vi "SS Class Init.vi"(7 "VI Refnum":refnum<vi>, 8 "error in (no error)":errorcluster, 9 "Init Data":variant, 10 "Device":string, 11 "Telescope in":refnum<class "Subsystem Telescope.lvclass">) -> (0 "error out":errorcluster, 2 "Channel List":refnum<class "HK Item.lvclass">[](array[class]), 3 "Telescope out":refnum<class "Subsystem Telescope.lvclass">)   [LabVIEW 2024, in "Subsystem Telescope.lvclass"]
uses:
  Subsystem Telescope.lvclass
  hk-channel-class/hk-channel-class/HK Item/HK Item.lvclass
  Subsystem Class.lvclass
  Telescope/Telescope.lvclass
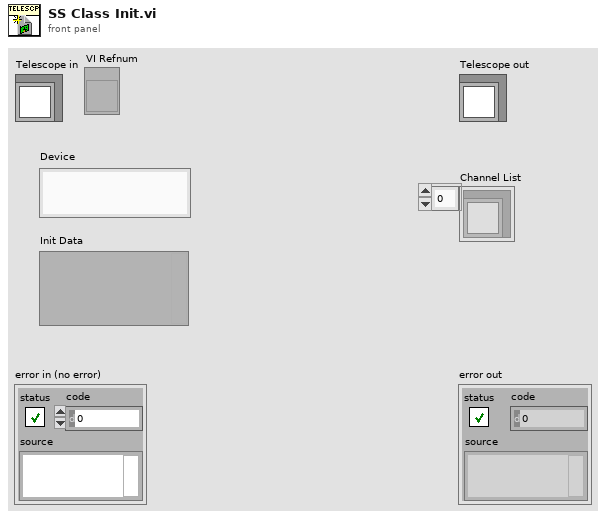
[diagram p1: front panel]
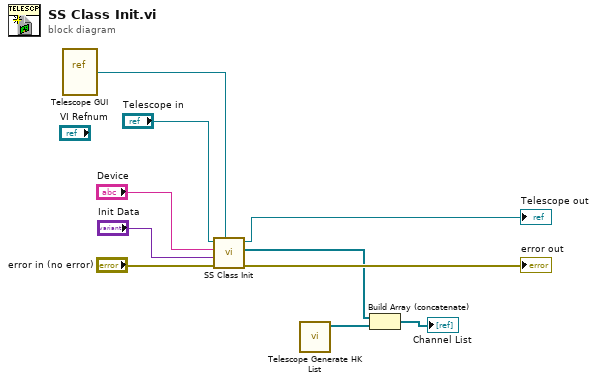
[diagram p0: block diagram]
diagram:
  n1 = vi-ref "Telescope GUI.vi"() -> (w4:refnum<vi>)
  n2 = call-parent "SS Class Init.vi"("VI Refnum"=w4, "error in (no error)"="error in (no error)", "Init Data"="Init Data", "Device"="Device", "Subsystem Class in"="Telescope in") -> ("error out"=→"error out":errorcluster, "Channel List"=w2:refnum<class "HK Item.lvclass">[], "Subsystem Class out"=→"Telescope out":refnum<class "Subsystem Telescope.lvclass">)  [unwired: 4 in]
  n3 = call "Telescope Generate HK List.vi"() -> ("Channel List"=w1:refnum<class "HK Item.lvclass">[])  [unwired: 10 in, 1 out]
  n4 = Build Array (concatenate)(w2, w1) -> (→"Channel List":refnum<class "HK Item.lvclass">[])
